vi "PID.vi"(10 "Right Setpoint":dbl, 11 "Left Setpoint":dbl) -> (0 "Right Setpoint (UI)":dbl, 1 "Left Setpoint (UI)":dbl, 2 "Right Setpoint (Motor)":dbl, 3 "Left Setpoint (Motor)":dbl)   [LabVIEW 2016]
uses:
  <vilib>/addons/control/pid/pid.llb/PID (DBL).vi
  <vilib>/addons/control/pid/NI_PID_pid.lvlib
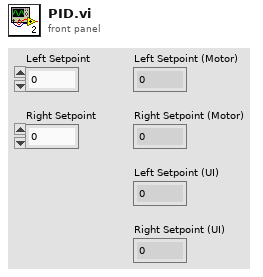
[diagram p1: front panel]
types:
  T1 = cluster{"proportional gain (Kc)":dbl, "integral time (Ti, min)":dbl, "derivative time (Td, min)":dbl}
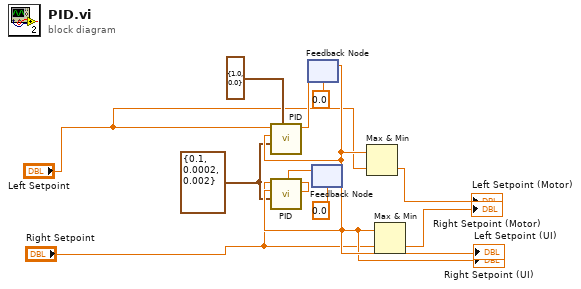
[diagram p0: block diagram]
diagram:
  w1 = T1 {"proportional gain (Kc)"=0.1, "integral time (Ti, min)"=0.0002, "derivative time (Td, min)"=0.002} ("PID gains")
  n1 = feedback #1(0.0 ("output")) -> (w12:dbl)
  "Left Setpoint (UI)" <- w12
  n2 = call-poly <vilib>:"PID.vi"("output range"=cluster{"output high":dbl, "output low":dbl} {"output high"=1.0, "output low"=0.0}, "PID gains"=w1, "process variable"=w12, "setpoint"="Left Setpoint") -> ("output"=w4:dbl)  [unwired: 6 in, 1 out]
  n3 = feedback-in #1(w4) -> ()
  n4 = feedback #2(0.0 ("output")) -> (w11:dbl)
  "Right Setpoint (UI)" <- w11
  n5 = call-poly <vilib>:"PID.vi"("PID gains"=w1, "process variable"=w11, "setpoint"="Right Setpoint") -> ("output"=w5:dbl)  [unwired: 7 in, 1 out]
  n6 = feedback-in #2(w5) -> ()
  n7 = Max & Min(x=w12, y="Left Setpoint") -> (min(x,y)=→"Left Setpoint (Motor)":dbl)  [unwired: 1 out]
  n8 = Max & Min(x=w11, y="Right Setpoint") -> (min(x,y)=→"Right Setpoint (Motor)":dbl)  [unwired: 1 out]
